vi "Growth_Info_Prompt.vi"(0 "Operator Name In":string, 1 "Growth Name In":string, 2 "Notes In":string) -> (3 "Operator Name Out":string, 4 "Growth Name Out":string, 5 "Notes Out":string, 6 "Cancelled":bool)   [LabVIEW 2011]
doc: "This VI prompts the user for the operator name, growth name, and any notes pertaining to the current growth sequence."
panel:
  in  "Notes":string
  in  "Cancel":bool
  in  "OK":bool
  in  "Growth Name":string
  in  "Operator Name":string
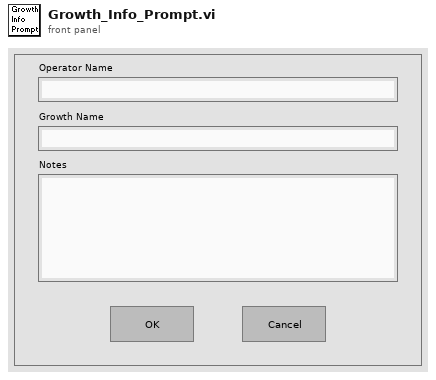
[diagram p1: front panel]
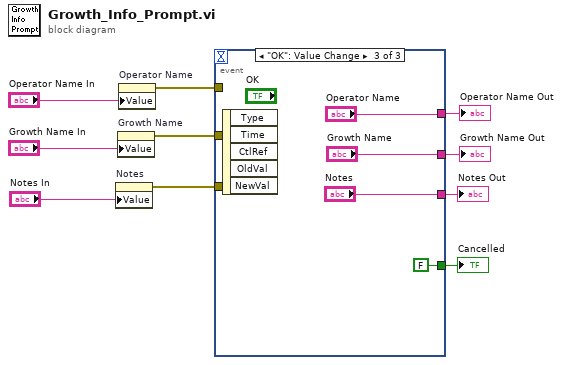
[diagram p0: block diagram]
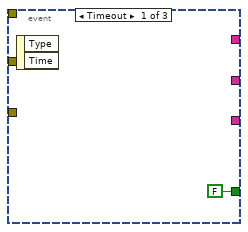
[diagram p2: hidden frame]
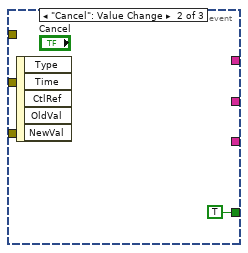
[diagram p3: hidden frame]
diagram:
  n1 = property on="Notes" class="Str"("Value"="Notes In") -> (error out=w4:errorcluster)  [unwired: 2 in, 1 out]
  n2 = property on="Growth Name" class="Str"("Value"="Growth Name In") -> (error out=w5:errorcluster)  [unwired: 2 in, 1 out]
  n3 = property on="Operator Name" class="Str"("Value"="Operator Name In") -> (error out=w6:errorcluster)  [unwired: 2 in, 1 out]
  n4 = event shown="[2] \"OK\": Value Change" {
    selector: _ -> [_ _ _]
    dyn-events: _ -> [_ _ _]
    timeout: _ -> [_ _ _]
    tunnel: [FALSE TRUE FALSE] -> w10
    tunnel: [_ _ "Operator Name"] -> w9
    tunnel: [_ _ "Growth Name"] -> w8
    tunnel: [_ _ "Notes"] -> w7
    tunnel: w6 -> [_ _ _]
    tunnel: w5 -> [_ _ _]
    tunnel: w4 -> [_ _ _]
    event Timeout {
      n5 = event-data() -> ()  [unwired: 1 in, 2 out]
    }
    event "Cancel": Value Change {
      n6 = event-data() -> ()  [unwired: 1 in, 5 out]
    }
    event "OK": Value Change {
      n7 = event-data() -> ()  [unwired: 1 in, 5 out]
    }
  }
  "Cancelled" <- w10
  "Notes Out" <- w7
  "Growth Name Out" <- w8
  "Operator Name Out" <- w9
